vi "Type Info Generation.vi"(8 "error in (no error)":errorcluster) -> (0 "error out":errorcluster)   [LabVIEW 2020]
uses:
  <vilib>/addons/_JKI Toolkits/Caraya/classes/Assert/Assert True.vi
  <vilib>/addons/_JKI Toolkits/Caraya/classes/Assert/Assert Equal Value and Type_Variant.vi
  <vilib>/addons/_JKI Toolkits/Caraya/classes/Assert/Assert Error.vi
  <vilib>/addons/_JKI Toolkits/Caraya/classes/Test/Test.lvclass
  G-Embedded-Python-Interpreter-Toolkit/G-Embedded-Python-Interpreter-Toolkit.lvlib
  <vilib>/addons/_JKI Toolkits/Caraya/classes/Assert/Assert.lvclass
  <vilib>/Utility/Data Type/Type Definitions/Data Type.ctl
  <vilib>/Utility/Data Type/NI_Data Type.lvlib
  G-Embedded-Python-Interpreter-Toolkit/Type Information.ctl
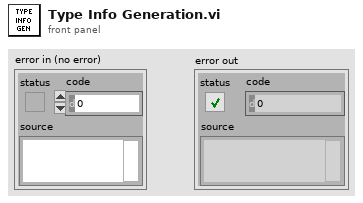
[diagram p1: front panel]
types:
  T1 = typedef "G-Embedded-Python-Interpreter-Toolkit.lvlib/Type Information.ctl" = cluster{"Type":T2, "Array Dimensions":u8}
  T2 = typedef "NI_Data Type.lvlib/Data Type.ctl" = enum8{"Invalid Type", "Void", "I8", "I16", "I32", "I64", "U8", "U16", "U32", "U64", "Single Float", "Double Float", "Extended Float", "Single Complex", "Double Complex", "Extended Complex", "Enum U8", "Enum U16", "Enum U32", "Enum U64", "Single Float With Unit", "Double Float With Unit", "Extended Float With Unit", "Single Complex with Unit", "Double Complex with Unit", "Extended Complex with Unit", "Boolean", "String", "Path", "Picture", "Tag", "Array", "Cluster", "Variant", "LV Variant", "Waveform", "Timestamp", "Digital Waveform", "Digital Data", "ExpressData", "Refnum", "External Data", "VI", "Poly VI", "LabVIEW Class Instance", "Fixed Point", "Set Collection", "Map Collection"}
  T3 = typedef "G-Embedded-Python-Interpreter-Toolkit.lvlib/Python Object Reference.ctl" = refnum<k1>
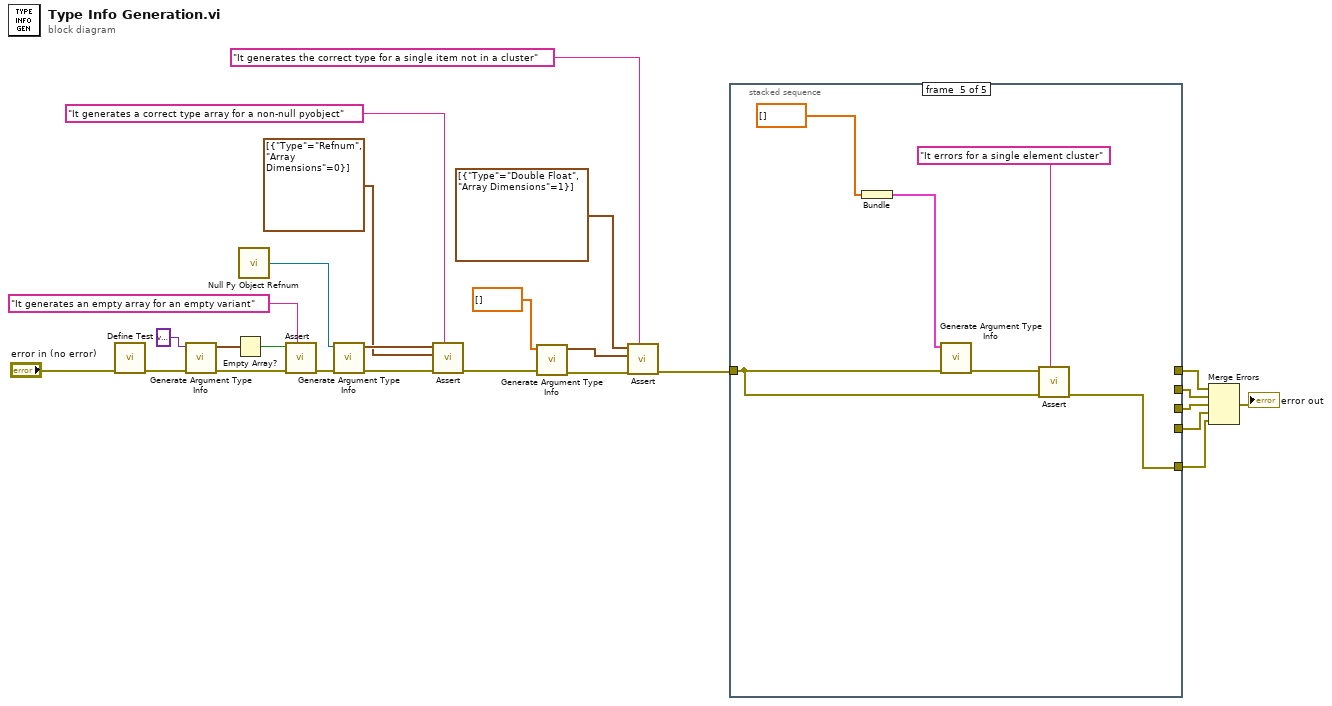
[diagram p0: block diagram]
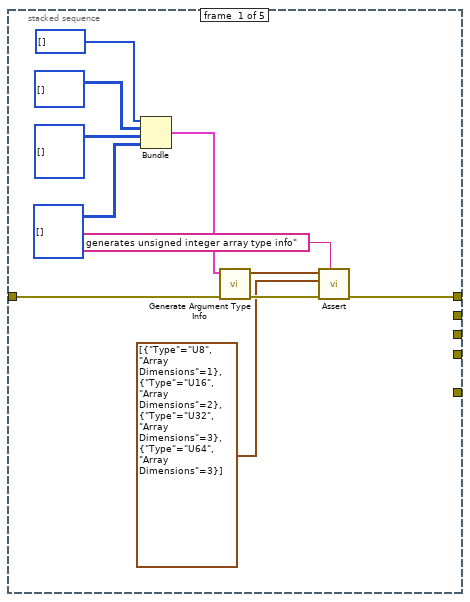
[diagram p2: hidden frame]
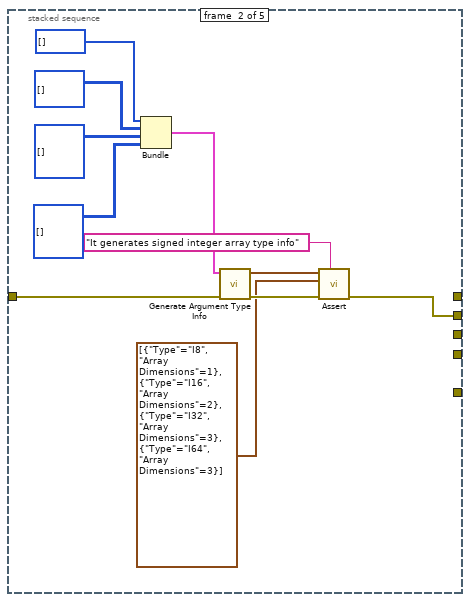
[diagram p3: hidden frame]
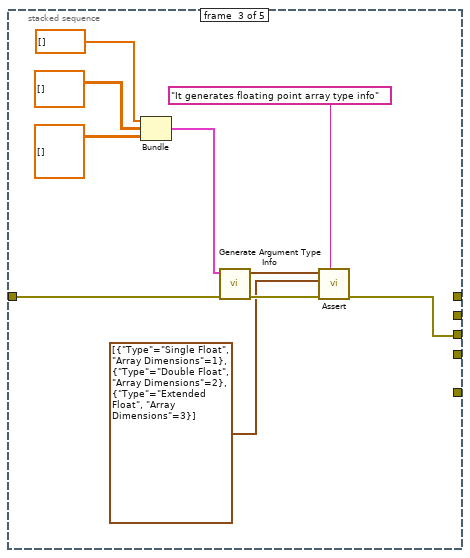
[diagram p4: hidden frame]
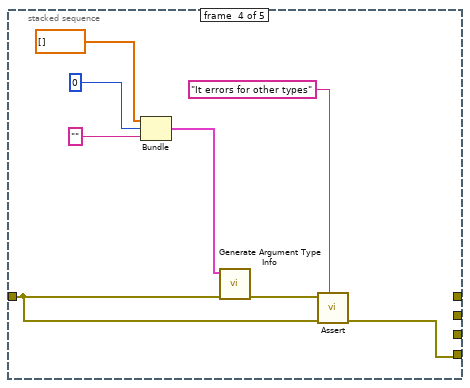
[diagram p5: hidden frame]
diagram:
  n1 = call <vilib>:"Define Test.vi"("error in (no error)"="error in (no error)") -> ("error out"=w25:errorcluster)  [unwired: 10 in]
  n2 = call "Generate Argument Type Info.vi"("error in (no error)"=w25, "Data Type"=variant) -> ("error out"=w22:errorcluster, "Array"=w24:T1[])  [unwired: 8 in]
  n3 = Empty Array?(array=w24) -> (empty?=w23:bool)
  n4 = call "Null Py Object Refnum.vi"() -> ("Null Python Object Refnum"=w9:T3)
  n5 = call-poly <vilib>:"Assert.vi"("Label"="It generates an empty array for an empty variant", "error in (no error)"=w22, "True?"=w23) -> ("error out"=w15:errorcluster)  [unwired: 8 in]
  n6 = call "Generate Argument Type Info.vi"("error in (no error)"=w15, "Data Type"=w9) -> ("error out"=w20:errorcluster, "Array"=w17:T1[])  [unwired: 8 in]
  n7 = call-poly <vilib>:"Assert.vi"("Label"="It generates a correct type array for a non-null pyobject", "error in (no error)"=w20, "Y"=T1[] [{"Type"=enum."Refnum", "Array Dimensions"=0}] ("Array"), "X"=w17) -> ("error out"=w7:errorcluster)  [unwired: 7 in]
  n8 = call "Generate Argument Type Info.vi"("error in (no error)"=w7, "Data Type"=dbl[] []) -> ("error out"=w6:errorcluster, "Array"=w4:T1[])  [unwired: 8 in]
  n9 = call-poly <vilib>:"Assert.vi"("Label"="It generates the correct type for a single item not in a cluster", "error in (no error)"=w6, "Y"=w4, "X"=T1[] [{"Type"=enum."Double Float", "Array Dimensions"=1}] ("Array")) -> ("error out"=w5:errorcluster)  [unwired: 7 in]
  n10 = stacked-sequence {
    tunnel: w5 -> [w37 w48 w58 w59 w68]
    tunnel: [w27 _ _ _ _] -> w14
    tunnel: [_ w38 _ _ _] -> w13
    tunnel: [_ _ w49 _ _] -> w12
    tunnel: [_ _ _ w61 _] -> w11
    tunnel: [_ _ _ _ w67] -> w8
    frame #0 {
      n11 = Bundle(u8[] [], u16[][] [], u32[][][] [], u64[][][] []) -> (w36:cluster{u8[], u16[][], u32[][][], u64[][][]})  [unwired: 1 in]
      n12 = call "Generate Argument Type Info.vi"("error in (no error)"=w37, "Data Type"=w36) -> ("error out"=w31:errorcluster, "Array"=w28:T1[])  [unwired: 8 in]
      n13 = call-poly <vilib>:"Assert.vi"("Label"="It generates unsigned integer array type info", "error in (no error)"=w31, "Y"=T1[] [{"Type"=enum."U8", "Array Dimensions"=1}, {"Type"=enum."U16", "Array Dimensions"=2}, {"Type"=enum."U32", "Array Dimensions"=3}, {"Type"=enum."U64", "Array Dimensions"=3}] ("Array"), "X"=w28) -> ("error out"=w27:errorcluster)  [unwired: 7 in]
    }
    frame #1 {
      n14 = Bundle(i8[] [], i16[][] [], i32[][][] [], i64[][][] []) -> (w47:cluster{i8[], i16[][], i32[][][], i64[][][]})  [unwired: 1 in]
      n15 = call "Generate Argument Type Info.vi"("error in (no error)"=w48, "Data Type"=w47) -> ("error out"=w42:errorcluster, "Array"=w39:T1[])  [unwired: 8 in]
      n16 = call-poly <vilib>:"Assert.vi"("Label"="It generates signed integer array type info", "error in (no error)"=w42, "Y"=T1[] [{"Type"=enum."I8", "Array Dimensions"=1}, {"Type"=enum."I16", "Array Dimensions"=2}, {"Type"=enum."I32", "Array Dimensions"=3}, {"Type"=enum."I64", "Array Dimensions"=3}] ("Array"), "X"=w39) -> ("error out"=w38:errorcluster)  [unwired: 7 in]
    }
    frame #2 {
      n17 = Bundle(sgl[] [], dbl[][] [], ext[][][] []) -> (w57:cluster{sgl[], dbl[][], ext[][][]})  [unwired: 1 in]
      n18 = call "Generate Argument Type Info.vi"("error in (no error)"=w58, "Data Type"=w57) -> ("error out"=w53:errorcluster, "Array"=w50:T1[])  [unwired: 8 in]
      n19 = call-poly <vilib>:"Assert.vi"("Label"="It generates floating point array type info", "error in (no error)"=w53, "Y"=T1[] [{"Type"=enum."Single Float", "Array Dimensions"=1}, {"Type"=enum."Double Float", "Array Dimensions"=2}, {"Type"=enum."Extended Float", "Array Dimensions"=3}] ("Array"), "X"=w50) -> ("error out"=w49:errorcluster)  [unwired: 7 in]
    }
    frame #3 {
      n20 = Bundle(csg[] [], 0, "") -> (w66:cluster{csg[], i32, string})  [unwired: 1 in]
      n21 = call "Generate Argument Type Info.vi"("error in (no error)"=w59, "Data Type"=w66) -> ("error out"=w60:errorcluster)  [unwired: 8 in, 1 out]
      n22 = call-poly <vilib>:"Assert.vi"("Label"="It errors for other types", "error in (no error)"=w59, "Error?"=w60) -> ("error out"=w61:errorcluster)  [unwired: 8 in]
    }
    frame #4 {
      n23 = Bundle(dbl[] []) -> (w72:cluster{dbl[]})  [unwired: 1 in]
      n24 = call "Generate Argument Type Info.vi"("error in (no error)"=w68, "Data Type"=w72) -> ("error out"=w69:errorcluster)  [unwired: 8 in, 1 out]
      n25 = call-poly <vilib>:"Assert.vi"("Label"="It errors for a single element cluster", "error in (no error)"=w68, "Error?"=w69) -> ("error out"=w67:errorcluster)  [unwired: 8 in]
    }
  }
  n26 = Merge Errors(w14, w13, w12, w11, w8) -> (→"error out":errorcluster)
